vi "Mini projek (Broncial).vi"() -> ()   [LabVIEW 2015]
uses:
  <vilib>/express/express analysis/Spectral/Block/exnSpectralBlock spectral measurements RMS poly.vi
  <vilib>/express/express analysis/Spectral/Block/exnSpectralBlock spectral measurements RMS DDT.vi
  <vilib>/express/express analysis/Spectral/XNode/ExpressSpectralMeasurementsBlockNode.xnode
  <vilib>/gmath/NI_Gmath.lvlib
panel:
  out "FFT":dynamicdata(graph)
  in  "Stop":bool
  out "Samples Read":i32
  out "Time Domain":waveform(dbl)[](graph)
  out "STFT Spectrogram":dbl[][](graph)
  in  "file path":path
  in  "number of samples/ch (-1: all)":i32=-1
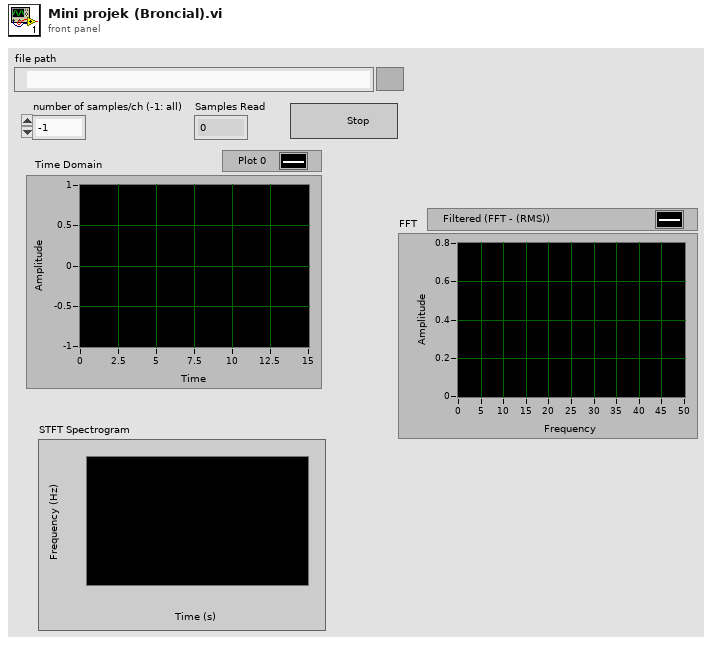
[diagram p1: front panel]
types:
  T1 = cluster{"averaging mode":u16, "weighting mode":u16, "number of averages":u32}
  T2 = cluster{"dB On (F)":bool, "unwrap phase (F)":bool, "convert to degree (F)":bool}
  T3 = cluster{"data[0]":waveform(dbl), "data[1]":waveform(dbl), "data[2]":waveform(dbl), "data[3]":waveform(dbl), "data[4]":waveform(dbl), "data[5]":waveform(dbl), "data[6]":waveform(dbl), "data[7]":waveform(dbl), "data[8]":waveform(dbl)}
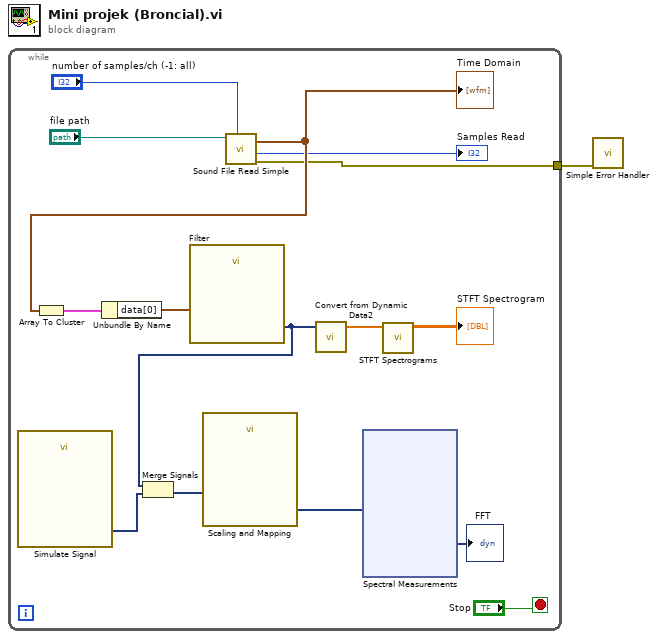
[diagram p0: block diagram]
diagram:
  n1 = while {
    tunnel: [w13] -> w1
    stop <- "Stop" stop-if-true
    n2 = call "Simulate Signal"() -> ("Sine with Uniform Noise"=w2:dynamicdata)  [unwired: 14 in, 1 out]
    n3 = call <vilib>:"Sound File Read Simple.vi"("number of samples/ch (-1: all)"="number of samples/ch (-1: all)", "path"="file path") -> ("error out"=w13:errorcluster, "offset"=→"Samples Read":i32, "data"=w15:waveform(dbl)[])  [unwired: 6 in, 1 out]
    "Time Domain" <- w15
    n4 = Array To Cluster(array=w15) -> (cluster=w11:T3)
    n5 = Unbundle By Name(w11) -> ("data[0]"=w7:waveform(dbl))
    n6 = call "Filter"("Signal"=w7) -> ("Filtered Signal"=w6:dynamicdata)  [unwired: 9 in, 1 out]
    n7 = Merge Signals(w6, w2) -> (w3:dynamicdata)
    n8 = call "Scaling and Mapping"("Signals"=w3) -> ("Scaled Signals"=w5:dynamicdata)  [unwired: 9 in, 1 out]
    n9 = call "Convert from Dynamic Data2"("Dynamic Data Type"=w6) -> ("Array"=w8:dbl[])  [unwired: 3 in]
    n10 = xnode "Spectral Measurements"("Signals"=w5) -> ("FFT - (RMS)"=→"FFT":dynamicdata)  [unwired: 1 in, 2 out]
    n11 = call <vilib>:"STFT Spectrograms.vi"("X"=w8) -> ("STFT Spectrogram {X}"=→"STFT Spectrogram":dbl[][])  [unwired: 9 in, 1 out]
  }
  n12 = call <vilib>:"Simple Error Handler.vi"("error in (no error)"=w1) -> ()  [unwired: 4 in, 5 out]
